vi "WPI_DMAAddChannelToStream_AnalogInput.vi"(7 "AIDeviceRef":T1={"DevStatus"={"status"=FALSE, "code"=0, "source"=""}, "Analog Channel"=enum."AI 1"}, 8 "error in (no error)":errorcluster, 10 "Analog Input Type":T3, 11 "DMARef":T4) -> (0 "error out":errorcluster, 3 "DMARef":T4)   [LabVIEW 2017]
doc: "Specifies the data transferred in the DMA stream. Wire a device reference from the other WPI Robotics Library Open VIs to specify the data you want to receive. The order that the AddChannel VIs add data to the DMA stream defines the order that the Read VI returns the data.\n\nSpecifies the analog input data transferred in the DMA stream.\n\nYou must open a reference to a DMA stream with the Open VI before using this VI.\n\nThis software is licensed. Open the labview\\readme\\WPI Robotics Library Open Source License.txt file for more information."
uses:
  <vilib>/Rock Robotics/WPI/DMA/WPI_DMARef.ctl
  <vilib>/Rock Robotics/WPI/DMA/WPI_DMAAnalogInputType.ctl
  <vilib>/Rock Robotics/WPI/AnalogChannel/WPI_AnalogChannelDevRef.ctl
  <vilib>/Rock Robotics/SystemInterfaces/AI/FPGA_AIChannel.ctl
  <vilib>/Rock Robotics/WPI/DMA/WPI_DMAChannelTypeEnum.ctl
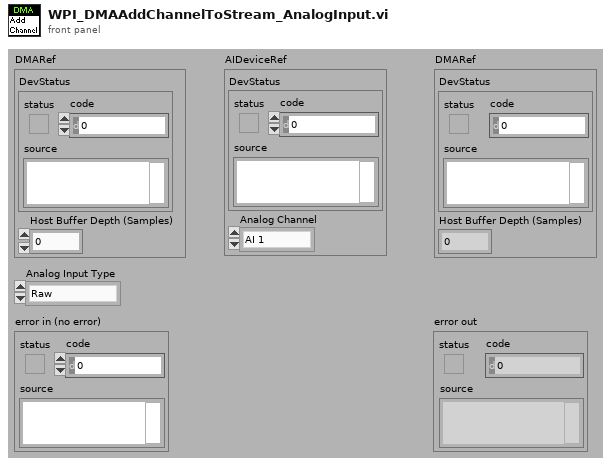
[diagram p1: front panel]
types:
  T1 = typedef "WPI_AnalogChannelDevRef.ctl" = cluster{"DevStatus":errorcluster, "Analog Channel":T2}
  T2 = typedef "FPGA_AIChannel.ctl" = enum8{"AI 0", "AI 1", "AI 2", "AI 3", "AI MXP 0", "AI MXP 1", "AI MXP 2", "AI MXP 3", "Invalid"}
  T3 = typedef "WPI_DMAAnalogInputType.ctl" = enum16{"Raw", "Averaged", "Accumulator"}
  T4 = typedef "WPI_DMARef.ctl" = cluster{"DevStatus":errorcluster, "Host Buffer Depth (Samples)":u32}
  T5 = typedef "WPI_DMAChannelTypeEnum.ctl" = enum16{"AI (Raw)", "AI (Avg)", "Accumulator", "DI (Raw) Onboard", "DI (Filtered) Onboard", "DI (Raw) MXP", "DI (Filtered) MXP", "Analog Trigger", "Counter", "Counter (Timer)", "Encoder", "Encoder (Timer)", "Time Stamp"}
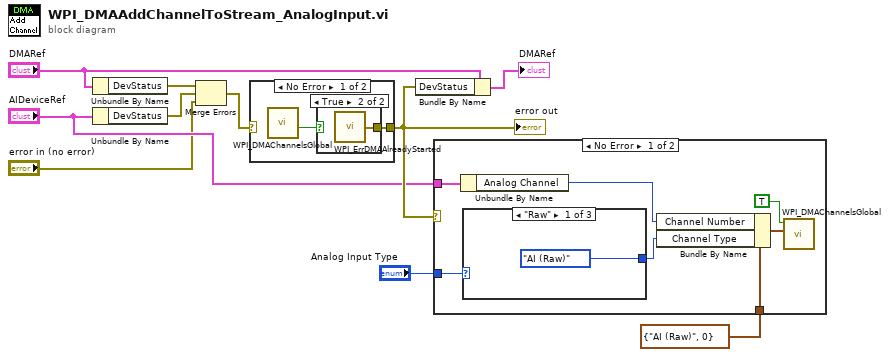
[diagram p0: block diagram]
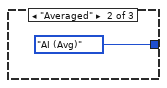
[diagram p2: hidden frame]
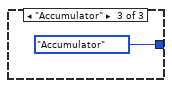
[diagram p3: hidden frame]
diagram:
  n1 = Unbundle By Name("DMARef") -> ("DevStatus"=w4:errorcluster)
  n2 = Unbundle By Name("AIDeviceRef") -> ("DevStatus"=w3:errorcluster)
  n3 = Merge Errors(w4, w3, "error in (no error)") -> (w1:errorcluster)
  n4 = case shown="No Error" w1 {
    selector: w1 -> [_ w14]
    tunnel: [w11 w14] -> w9
    frame No Error {
      n5 = call <vilib>:"WPI_DMAChannelsGlobal.vi"() -> ("Started"=w12:bool)  [unwired: 4 in, 7 out]
      n6 = case shown="True" w12 {
        tunnel: [_ w13] -> w11
        frame False {
        }
        frame True {
          n7 = call <vilib>:"WPI_ErrDMAAlreadyStarted.vi"() -> ("error out"=w13:errorcluster)
        }
      }
    }
    frame Error {
    }
  }
  "error out" <- w9
  n8 = Bundle By Name(cluster="DMARef", "DevStatus"=w9) -> (→"DMARef":T4)
  n9 = case shown="No Error" w9 {
    tunnel: "AIDeviceRef" -> [w20 _]
    tunnel: cluster{"Channel Type":T5, "Channel Number":u8} {"Channel Type"=enum."AI (Raw)", "Channel Number"=0} ("Channel") -> [w19 _]
    tunnel: "Analog Input Type" -> [w15 _]
    frame No Error {
      n10 = Unbundle By Name(w20) -> ("Analog Channel"=w16:T2)
      n11 = case shown="\"Raw\"" w15 {
        tunnel: [WPI_DMAChannelTypeEnum."AI (Raw)" ("Channel Type") WPI_DMAChannelTypeEnum."AI (Avg)" ("Channel Type") WPI_DMAChannelTypeEnum."Accumulator" ("Channel Type")] -> w17
        frame "Raw" {
        }
        frame "Averaged" {
        }
        frame "Accumulator" {
        }
      }
      n12 = Bundle By Name(cluster=w19, "Channel Number"=w16, "Channel Type"=w17) -> (w18:cluster{"Channel Type":T5, "Channel Number":u8})
      n13 = call <vilib>:"WPI_DMAChannelsGlobal.vi"("Channel"=w18, "Add"=TRUE) -> ()  [unwired: 2 in, 8 out]
    }
    frame Error {
    }
  }
